vi "Read Temp_Humi Example.vi"() -> ()   [LabVIEW 2016, in "Environment Chamber.lvlib" / "Climatic Chamber.lvlib"]
doc: "Basic Example to <b>monitor</b> the actual <b>Temperature and Humidity</b>."
uses:
  Climatic Chamber.lvlib
panel:
  out "New Data":bool
  in  "stop":bool
  out "Humidity":dbl(slide) scale=0.0..100.0
  out "Temperature":dbl(slide) scale=0.0..100.0
  in  "VISA resource name":refnum<visa-resource-name>="COM4"
  in  "Serial Configuration":T1={"Baud Rate"=19200, "Parity"=0, "Data Bits"=8, "Stop Bits"=10, "Flow Control"=0} {"Baud Rate" items=["300"=300, "600"=600, "1200"=1200, "2400"=2400, "4800"=4800, "9600"=9600, "19200"=19200]; "Parity" items=["None", "Odd", "Even", "Mark", "Space"]; "Data Bits" items=["7"=7, "8"=8]; "Stop Bits" items=["1.0"=10, "1.5"=15, "2.0"=20]; "Flow Control" items=["None", "XON/XOFF", "RTS/CTS", "XON/XOFF & RTS/CTS", "DTR/DSR", "XON/XOFF & DTR/DSR"]}
  out "Instrument Firmware Revision":string
  # "Serial settings"
  # "1. Enter Serial Port settings\nthat matches the settings in\nyour chamber\n\n2. In the Chambers\nCommunication Setup use\nCR+LF as delimiter and \nProtocol as STD\n \n3. Run the VI"
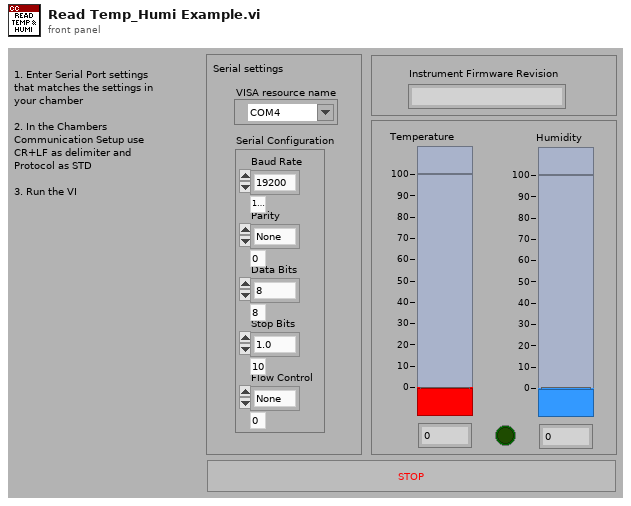
[diagram p1: front panel]
types:
  T1 = cluster{"Baud Rate":u32, "Parity":u16, "Data Bits":u16, "Stop Bits":u16, "Flow Control":u16}
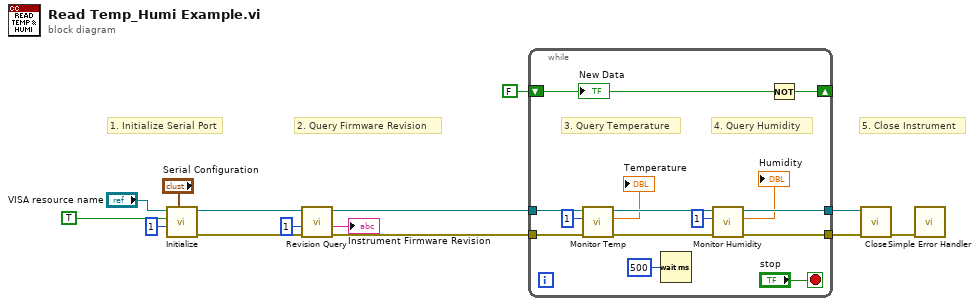
[diagram p0: block diagram]
diagram:
  # "5. Close Instrument"
  # "2. Query Firmware Revision"
  # "1. Initialize Serial Port"
  n1 = call "Initialize.vi"("Serial Configuration"="Serial Configuration", "Address (0)"=1, "ID Query (True)"=TRUE, "VISA resource name"="VISA resource name") -> ("error out"=w9:errorcluster, "VISA resource name out"=w10:refnum<visa-resource-name>)  [unwired: 6 in]
  n2 = call "Revision Query.vi"("error in (no error)"=w9, "Address (0)"=1, "VISA resource name"=w10) -> ("error out"=w8:errorcluster, "Instrument Firmware Revision"=→"Instrument Firmware Revision":string, "VISA resource name out"=w7:refnum<visa-resource-name>)  [unwired: 5 in, 1 out]
  n3 = while {
    tunnel: w8 -> [w27]
    tunnel: w7 -> [w26]
    tunnel: [w24] -> w4
    tunnel: [w22] -> w3
    shift-right: [w15] -> _
    shift-left: FALSE -> [w16]
    stop <- "stop" stop-if-true
    # "4. Query Humidity"
    # "3. Query Temperature"
    n4 = call "Monitor Temp.vi"("error in (no error)"=w27, "Address (0)"=1, "VISA resource name"=w26) -> ("error out"=w25:errorcluster, "measured temp"=→"Temperature":dbl, "VISA resource name out"=w23:refnum<visa-resource-name>)  [unwired: 3 in, 3 out]
    n5 = Wait (ms)(milliseconds to wait=u32 500) -> ()  [unwired: 1 out]
    n6 = call "Monitor Humidity.vi"("error in (no error)"=w25, "Address (0)"=1, "VISA resource name"=w23) -> ("error out"=w24:errorcluster, "measured humidity"=→"Humidity":dbl, "VISA resource name out"=w22:refnum<visa-resource-name>)  [unwired: 3 in, 3 out]
    n7 = Not(x=w16) -> (.not. x?=w15:bool)
    "New Data" <- w16
  }
  n8 = call "Close.vi"("error in (no error)"=w4, "VISA resource name"=w3) -> ("error out"=w2:errorcluster)  [unwired: 9 in]
  n9 = call <vilib>:"Simple Error Handler.vi"("error in (no error)"=w2) -> ()  [unwired: 4 in, 5 out]
